vi "Set Voltage and Current.vi"(0 "Yokogawa WT2X0 in":refnum<class "Yokogawa WT2X0.lvclass">, 5 "Card #":u8, 7 "Voltage enum number":u16, 9 "Current enum number":u16, 11 "error in (no error)":errorcluster) -> (4 "Yokogawa WT2X0 out":refnum<class "Yokogawa WT2X0.lvclass">, 15 "error out":errorcluster)   [LabVIEW 2014, in "Generic Power Analyzer.lvlib" / "Yokogawa WT2X0.lvlib" / "Yokogawa WT2X0.lvclass"]
uses:
  Yokogawa WT2X0.lvclass
  <instrlib>/Yokogawa WT200 Series/Yokogawa WT200 Series.lvlib
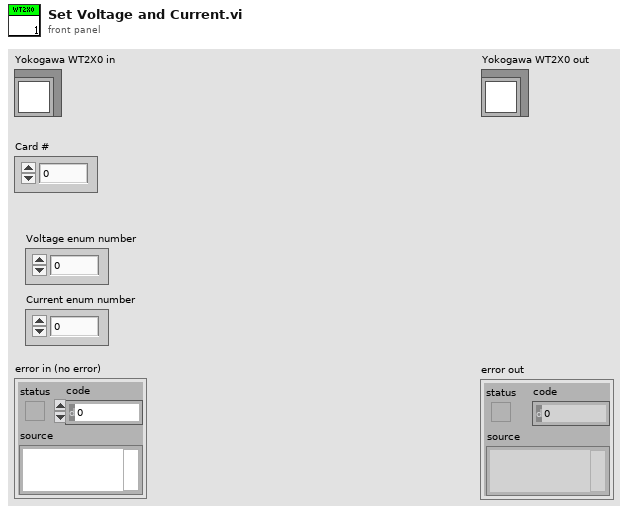
[diagram p1: front panel]
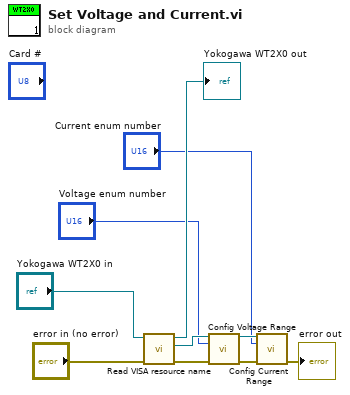
[diagram p0: block diagram]
diagram:
  n1 = call-dynamic "Read VISA resource name.vi"("error in (no error)"="error in (no error)", "Generic Instrument in"="Yokogawa WT2X0 in") -> ("error out"=w4:errorcluster, "VISA resource name"=w6:refnum<visa-resource-name>, "Generic Instrument out"=→"Yokogawa WT2X0 out":refnum<class "Yokogawa WT2X0.lvclass">)  [unwired: 7 in]
  n2 = call <instrlib>:"Config Voltage Range.vi"("VISA resource name"=w6, "V Range (6: 600V)"="Voltage enum number", "error in (no error)"=w4) -> ("VISA resource name out"=w10:refnum<visa-resource-name>, "error out"=w9:errorcluster)  [unwired: 11 in]
  n3 = call <instrlib>:"Config Current Range.vi"("VISA resource name"=w10, "A Range (12: 20A)"="Current enum number", "error in (no error)"=w9) -> ("error out"=→"error out":errorcluster)  [unwired: 11 in, 1 out]
